vi "Create.vi"(5 "Code Inspector in":refnum<class "Code Inspector.lvclass">, 8 "error in (no error)":errorcluster, 11 "Application":refnum<vi>) -> (0 "error out":errorcluster, 3 "Code Inspector":refnum<class "Code Inspector.lvclass">)   [LabVIEW 2017, in "Cobertura.lvlib" / "Code Inspector.lvclass"]
uses:
  Code Inspector.lvclass
  Code Inspector.lvclass/Code Inspector.ctl
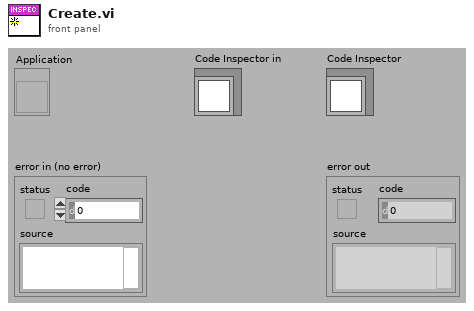
[diagram p1: front panel]
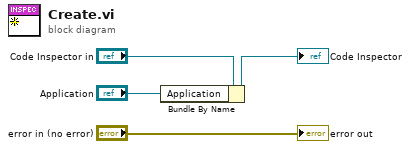
[diagram p0: block diagram]
diagram:
  n1 = Bundle By Name(cluster="Code Inspector in", "Application"="Application") -> (→"Code Inspector":refnum<class "Code Inspector.lvclass">)
  "error out" <- "error in (no error)"
